vi "Scale Type.vi"(8 "error in (no error)":errorcluster, 11 "Scale in":refnum<class "Scale Config.lvclass">) -> (0 "error out":errorcluster, 2 "Scale Type":T1, 3 "Scale out":refnum<class "Scale Config.lvclass">)   [LabVIEW 2023, in "VolatusConfig.lvlib" / "Scale Config.lvclass"]
uses:
  Scale Config.lvclass
  Scale Type.ctl
  VolatusConfigElement/VolatusConfigElement.lvclass/VolatusConfigElement.ctl
  VolatusConfigElement/Element.vi
  Scale Config.lvclass/Scale Config.ctl
  VolatusConfigElement/VolatusConfigElement.lvclass
  lv-cdm/CDM-Config/Config Element/Config Element.lvclass
  VolatusConfig.lvlib
  C:/dev/volatus/mts-volatus-super/libs/lv-volatus/VolatusConfig/VolatusConfigElement/VolatusConfigElement.lvclass
  C:/dev/volatus/mts-volatus-super/libs/lv-volatus/VolatusConfig/Scale/Scale Config.lvclass
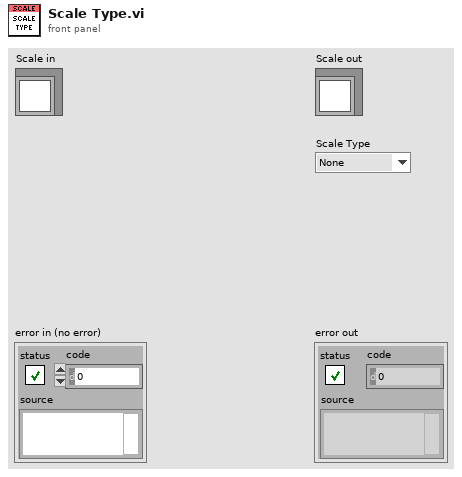
[diagram p1: front panel]
types:
  T1 = typedef "VolatusConfig.lvlib/Scale Type.ctl" = enum16{"None", "Sensor", "Polynomial", "Threshold", "Invert Bool", "Exponential"}
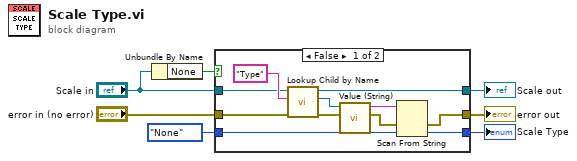
[diagram p0: block diagram]
diagram:
  n1 = Unbundle By Name("Scale in") -> ("None"=w1:bool)
  n2 = case shown="False" w1 {
    tunnel: [w13 w19] -> w7
    tunnel: "error in (no error)" -> [w12 w20]
    tunnel: [w11 w20] -> w5
    tunnel: [w10 w21] -> w4
    tunnel: "Scale in" -> [w9 w21]
    tunnel: Scale_Type."None" ("Scaling Type") -> [w8 w19]
    frame False {
      n3 = call "Lookup Child by Name.vi"("error in (no error)"=w12, "Child Name"="Type", "VolatusConfigElement in"=w9) -> ("error out"=w17:errorcluster, "Child"=w16:refnum<class "Config Element.lvclass">, "VolatusConfigElement out"=w10:refnum<class "Scale Config.lvclass">)  [unwired: 5 in, 1 out]
      n4 = call "Value (String).vi"("error in (no error)"=w17, "Config Element in"=w16) -> ("error out"=w14:errorcluster, "String Value"=w15:string)  [unwired: 8 in]
      n5 = Scan From String(input string=w15, error in=w14, default 1=w8) -> (error out=w11:errorcluster, output 1=w13:T1)  [unwired: 2 in, 2 out]
    }
    frame True {
    }
  }
  "error out" <- w5
  "Scale out" <- w4
  "Scale Type" <- w7
